vi "Autofocus.vi"(0 "Filter Type":T2(ring)=enum."Sobel", 1 "SpeedXY (mm/s)":dbl=100.0, 5 "X":dbl, 7 "Y":dbl, 9 "Z":dbl, 11 "error in (no error)":errorcluster, 12 "SpeedZ (mm/s)":dbl=10.0) -> (10 "Best Z value":string, 15 "error out":errorcluster)   [LabVIEW 2019]
uses:
  <vilib>/userDefined/High Color/IMAQdx.ctl
  <vilib>/vision/NI_Vision_Development_Module.lvlib
panel:
  out "Image 2":T1(plugin-control)
  out "Image 3":T1(plugin-control)
  in  "Stop":bool
  out "Last Z, mean and standard deviation:":string
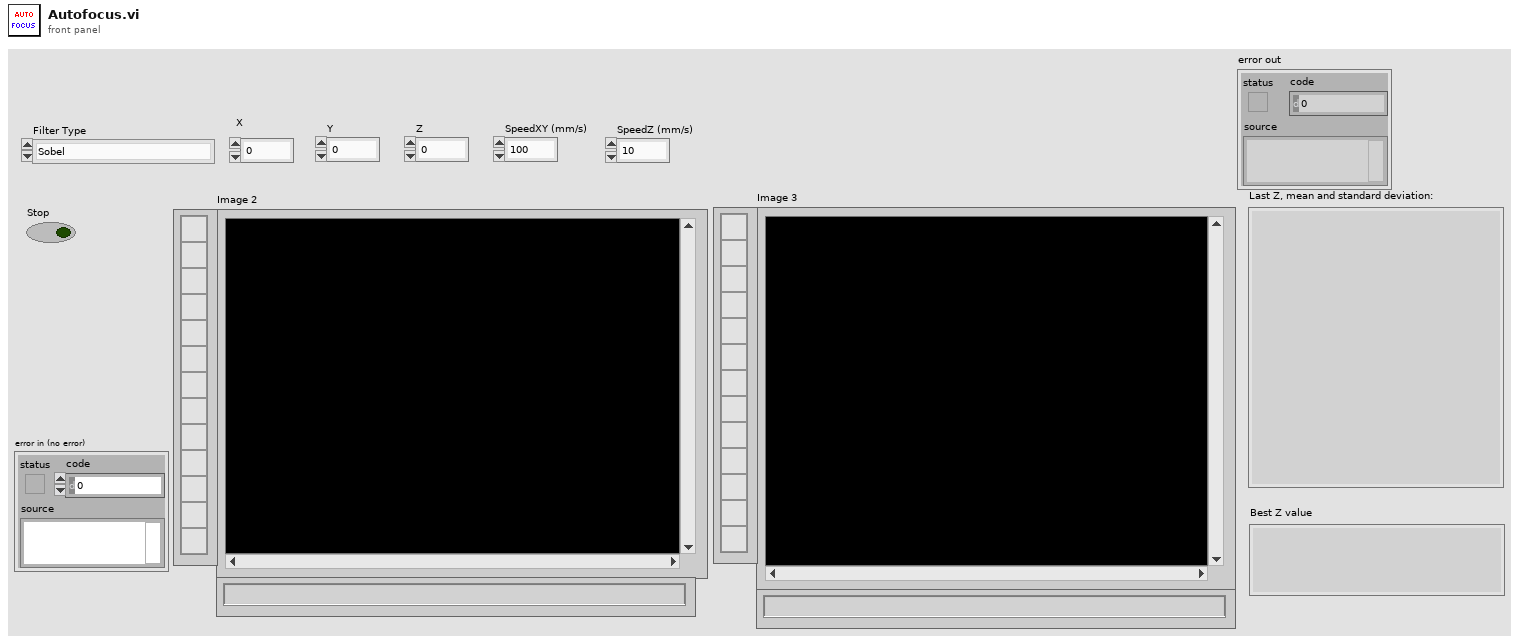
[diagram p1: front panel]
types:
  T1 = typedef "IMAQ Image.ctl" = refnum<image>
  T2 = enum16{"Convolution", "Differentiation", "Gradient", "Prewitt", "Roberts", "Sigma", "Sobel"}
  T3 = typedef "IMAQdx.ctl" = refnum<k21>
  T4 = enum32{"Differentiation", "Gradient", "Prewitt", "Roberts", "Sigma", "Sobel"}
  T5 = typedef "Image Type" = u32
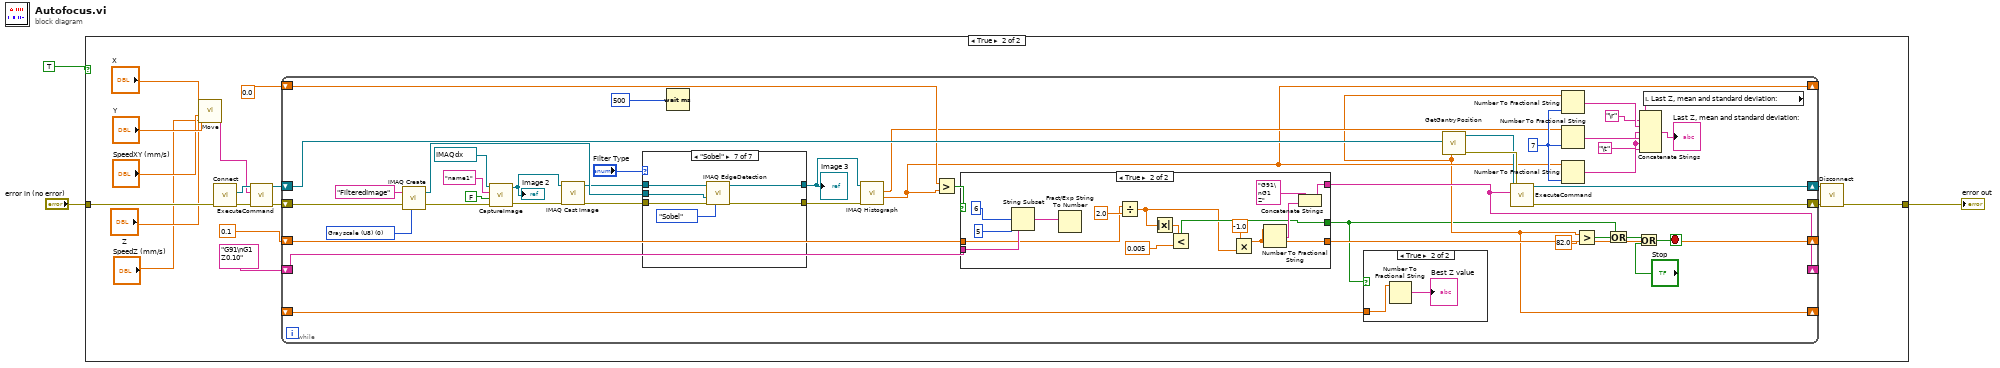
[diagram p0: block diagram]
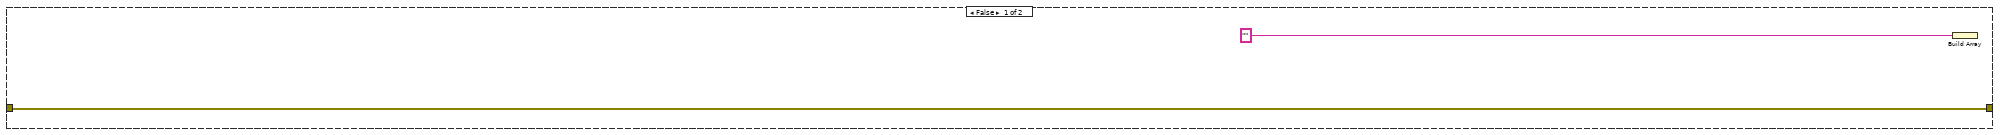
[diagram p2: hidden frame]
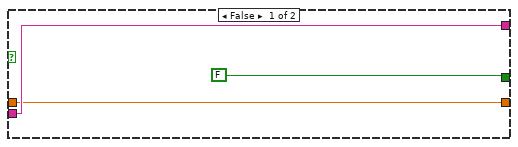
[diagram p4: hidden frame]
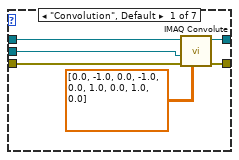
[diagram p5: hidden frame]
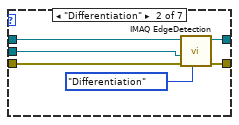
[diagram p6: hidden frame]
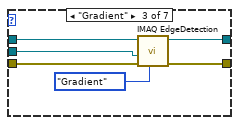
[diagram p7: hidden frame]
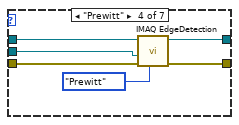
[diagram p8: hidden frame]
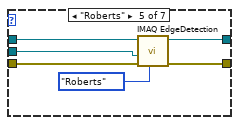
[diagram p9: hidden frame]
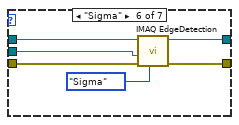
[diagram p10: hidden frame]
diagram:
  n1 = case shown="True" TRUE {
    tunnel: [w5 w16] -> w3
    tunnel: "error in (no error)" -> [w5 w15]
    frame False {
      n2 = Build Array("") -> ()  [unwired: 1 out]
    }
    frame True {
      n3 = call "Move.vi"("X"="X", "Y"="Y", "Z"="Z", "SpeedXY (mm/s)"="SpeedXY (mm/s)", "SpeedZ (mm/s)"="SpeedZ (mm/s)") -> ("Position Gcode"=w6:string)  [unwired: 10 in]
      n4 = call "Connect.vi"("error in (no error)"=w15) -> ("error out"=w19:errorcluster, "controller"=w20:refnum<k24>)  [unwired: 9 in]
      n5 = call "ExecuteCommand.vi"("error in (no error)"=w19, "Command Code"=w6, "controller in"=w20) -> ("error out"=w18:errorcluster, "controller out"=w17:refnum<k24>)  [unwired: 6 in, 1 out]
      n6 = while {
        shift-right: [w37] -> w22
        shift-left: w17 -> [w41]
        shift-right: [w39] -> w21
        shift-left: w18 -> [w59]
        shift-right: [w32] -> _
        shift-left: "G91\nG1 Z0.10" -> [w31]
        shift-right: [w26] -> _
        shift-left: 0.0 -> [w35]
        shift-right: [w28] -> _
        shift-left: 0.1 -> [w27]
        shift-right: [w25] -> _
        shift-left: _ -> [w24]
        stop <- w49 stop-if-true
        w51 = "\t"
        w55 = i16 7 ("precision (6)")
        w60 = T5 0 items=["Grayscale (U8)", "Grayscale (I16)", "Grayscale (SGL)", "Complex (CSG)", "RGB (U32)", "HSL (U32)", "RGB (U64)", "Grayscale (U16)"] ("Image Type")
        n7 = call "IMAQ Create"("Image Name"="FilteredImage", "Image Type"=w60, "error in (no error)"=w59) -> ("New Image"=w63:T1, "error out"=w62:errorcluster)  [unwired: 2 in]
        n8 = call "CaptureImage.vi"("Camera"=T3 "cam0", "ImageName"="name1", "Draw50MicroCircleAtCenter"=FALSE, "error in (no error)"=w62) -> ("Image"=w48:T1, "error out"=w47:errorcluster)  [unwired: 3 in]
        "Image 2" <- w48
        n9 = call "IMAQ Cast Image"("error in (no error)"=w47, "Image Src"=w48) -> ("error out"=w46:errorcluster, "Image Dst Out"=w45:T1)  [unwired: 8 in]
        n10 = case shown="\"Sobel\"" "Filter Type" {
          tunnel: w45 -> [w92 w98 w104 w110 w116 w122 w128]
          tunnel: w46 -> [w91 w97 w103 w109 w115 w121 w127]
          tunnel: w63 -> [w90 w99 w105 w111 w117 w123 w129]
          tunnel: [w89 w94 w100 w106 w112 w118 w124] -> w56
          tunnel: [w88 w95 w101 w107 w113 w119 w125] -> w57
          frame "Convolution", Default {
            n11 = call "IMAQ Convolute"("Kernel"=sgl[][] [[0.0, -1.0, 0.0], [-1.0, 0.0, 1.0], [0.0, 1.0, 0.0]], "error in (no error)"=w91, "Image Dst"=w90, "Image Src"=w92) -> ("error out"=w89:errorcluster, "Image Dst Out"=w88:T1)  [unwired: 6 in]
          }
          frame "Differentiation" {
            n12 = call "IMAQ EdgeDetection"("Method"=T4."Differentiation", "error in (no error)"=w97, "Image Dst"=w99, "Image Src"=w98) -> ("error out"=w94:errorcluster, "Image Dst Out"=w95:T1)  [unwired: 6 in]
          }
          frame "Gradient" {
            n13 = call "IMAQ EdgeDetection"("Method"=T4."Gradient", "error in (no error)"=w103, "Image Dst"=w105, "Image Src"=w104) -> ("error out"=w100:errorcluster, "Image Dst Out"=w101:T1)  [unwired: 6 in]
          }
          frame "Prewitt" {
            n14 = call "IMAQ EdgeDetection"("Method"=T4."Prewitt", "error in (no error)"=w109, "Image Dst"=w111, "Image Src"=w110) -> ("error out"=w106:errorcluster, "Image Dst Out"=w107:T1)  [unwired: 6 in]
          }
          frame "Roberts" {
            n15 = call "IMAQ EdgeDetection"("Method"=T4."Roberts", "error in (no error)"=w115, "Image Dst"=w117, "Image Src"=w116) -> ("error out"=w112:errorcluster, "Image Dst Out"=w113:T1)  [unwired: 6 in]
          }
          frame "Sigma" {
            n16 = call "IMAQ EdgeDetection"("Method"=T4."Sigma", "error in (no error)"=w121, "Image Dst"=w123, "Image Src"=w122) -> ("error out"=w118:errorcluster, "Image Dst Out"=w119:T1)  [unwired: 6 in]
          }
          frame "Sobel" {
            n17 = call "IMAQ EdgeDetection"("Method"=T4."Sobel", "error in (no error)"=w127, "Image Dst"=w129, "Image Src"=w128) -> ("error out"=w124:errorcluster, "Image Dst Out"=w125:T1)  [unwired: 6 in]
          }
        }
        "Image 3" <- w57
        n18 = Wait (ms)(milliseconds to wait=500) -> ()  [unwired: 1 out]
        n19 = call "IMAQ Histograph"("error in (no error)"=w56, "Image"=w57) -> ("Standard  Deviation"=w26:sgl, "Mean Value"=w34:sgl)  [unwired: 6 in, 2 out]
        n20 = Greater?(x=w35, y=w26) -> (0:w33:bool)
        n21 = case shown="True" w33 {
          tunnel: [w72 w86] -> w32
          tunnel: w31 -> [w72 w80]
          tunnel: [FALSE w81] -> w23
          tunnel: [w70 w76] -> w28
          tunnel: w27 -> [w70 w75]
          frame False {
          }
          frame True {
            n22 = String Subset(string=w80, offset (0)=6, length (rest)=5) -> (substring=w77:string)
            n23 = Fract/Exp String To Number(string=w77) -> ()  [unwired: 3 in, 2 out]
            n24 = Divide(x=w75, y=2.0) -> (x/y=w74:dbl)
            n25 = Absolute Value(x=w74) -> (abs(x)=w73:dbl)
            n26 = Less?(x=w73, y=0.005) -> (x < y?=w81:bool)
            n27 = Multiply(x=-1.0, y=w74) -> (x*y=w76:dbl)
            n28 = Number To Fractional String(number=w76) -> (F-format string=w85:string)  [unwired: 3 in]
            n29 = Concatenate Strings("G91\nG1 Z", w85) -> (w86:string)
          }
        }
        n30 = case shown="True" w23 {
          tunnel: w24 -> [_ w68]
          frame False {
          }
          frame True {
            n31 = Number To Fractional String(number=w68) -> (F-format string=→"Best Z value":string)  [unwired: 3 in]
          }
        }
        n32 = call "GetGantryPosition.vi"("Controller In"=w41) -> ("error out"=w40:errorcluster, "controller out"=w38:refnum<k24>, "Position Z"=w25:dbl)  [unwired: 4 in, 4 out]
        n33 = call "ExecuteCommand.vi"("error in (no error)"=w40, "Command Code"=w32, "controller in"=w38) -> ("error out"=w39:errorcluster, "controller out"=w37:refnum<k24>)  [unwired: 6 in, 1 out]
        n34 = Number To Fractional String(number=w25, precision (6)=w55) -> (F-format string=w54:string)  [unwired: 2 in]
        n35 = Number To Fractional String(number=w34, precision (6)=w55) -> (F-format string=w53:string)  [unwired: 2 in]
        n36 = Number To Fractional String(number=w26, precision (6)=w55) -> (F-format string=w52:string)  [unwired: 2 in]
        n37 = Greater?(x=w25, y=82.0) -> (0:w30:bool)
        n38 = Or(x=w30, y=w23) -> (x .or. y?=w29:bool)
        n39 = Or(x=w29, y="Stop") -> (x .or. y?=w49:bool)
        n40 = local read "Last Z, mean and standard deviation:"() -> (w44:string)
        n41 = Concatenate Strings(w44, "\r", w54, w51, w53, w51, w52) -> (→"Last Z, mean and standard deviation:":string)
      }
      n42 = call "Disconnect.vi"("error in (no error)"=w21, "controller"=w22) -> ("error out"=w16:errorcluster)  [unwired: 9 in]
    }
  }
  "error out" <- w3
